vi "Handle Errors.vi"(8 "error in":errorcluster, 11 "cCRDS_new in":refnum<class "cCRDS.lvclass">=refnum) -> (0 "error out":errorcluster, 2 "errors":errorcluster[](array[cluster]), 3 "cCRDS_new out":refnum<class "cCRDS.lvclass">)   [LabVIEW 2015, in "cCRDS.lvclass"]
uses:
  cCRDS.lvclass
  Reusable/CRDS/Main/CRDS.lvclass
  Reusable/Instrument/Instrument.lvclass
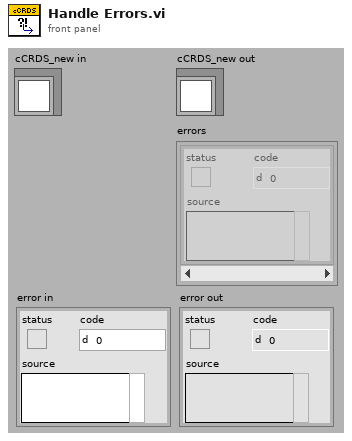
[diagram p1: front panel]
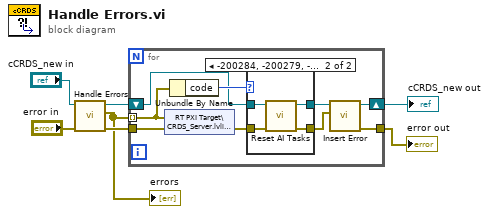
[diagram p0: block diagram]
diagram:
  n1 = call-parent "Handle Errors.vi"("error in"="error in", "Instrument in"="cCRDS_new in") -> ("error out"=w4:errorcluster, "errors"=w3:errorcluster[], "Instrument out"=w5:refnum<class "cCRDS.lvclass">)  [unwired: 7 in]
  "errors" <- w3
  n2 = for {
    tunnel: w3 -> [w10] mode=indexing
    shift-right: [w12] -> w2
    shift-left: w5 -> [w15]
    tunnel: w4 -> [w9]
    tunnel: [w11] -> w1
    n3 = shared-variable "RT PXI Target\\CRDS_Server.lvlib\\error"(w10, error in=w9) -> (error out=w8:errorcluster)
    n4 = Unbundle By Name(w10) -> ("code"=w16:i32)
    n5 = case shown="-200284, -200279, -200222, -200019" w16 {
      tunnel: w15 -> [w18 w22]
      tunnel: [w18 w19] -> w14
      tunnel: w8 -> [w17 w21]
      tunnel: [w17 w20] -> w13
      frame 0, Default {
      }
      frame -200284, -200279, -200222, -200019 {
        n6 = call "Reset AI Tasks.vi"("error in"=w21, "cCRDS in"=w22) -> ("error out"=w20:errorcluster, "cCRDS out"=w19:refnum<class "cCRDS.lvclass">)  [unwired: 8 in]
      }
    }
    n7 = call "Insert Error.vi"("err"=w13, "Instrument in"=w14) -> ("error out"=w11:errorcluster, "Instrument out"=w12:refnum<class "cCRDS.lvclass">)  [unwired: 7 in, 1 out]
  }
  "error out" <- w1
  "cCRDS_new out" <- w2
